vi "openOutput.vi"(8 "error in (no error)":errorcluster, 11 "DIO64Output in":refnum<class "DIO64Output.lvclass">) -> (0 "error out":errorcluster, 3 "DIO64Output out":refnum<class "DIO64Output.lvclass">)   [LabVIEW 2011, in "Hardware.lvlib" / "Channels.lvlib" / "DIO64Output.lvclass"]
doc: "Abstract Method.\n\nShould be overwritten by implementation of a digital output channel which require special treatment to initialise the channel.\n\nFor example, the Dio64 card require it to be opened and loaded, and kept in this state the whole time it is in use."
uses:
  DIO64Output.lvclass
  DIO64Output.lvclass/DIO64Output.ctl
  Channels.lvlib
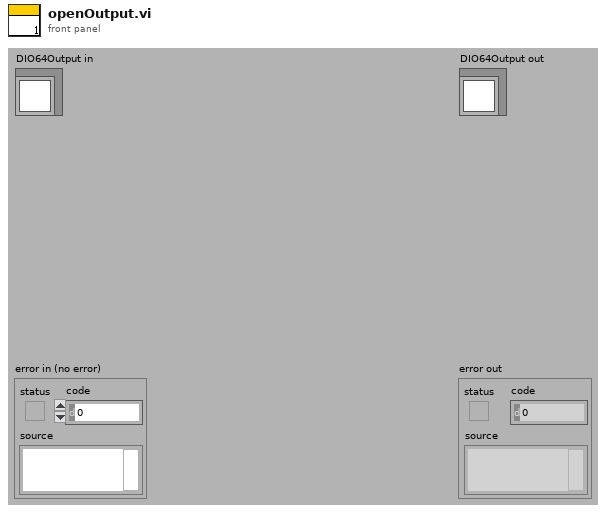
[diagram p1: front panel]
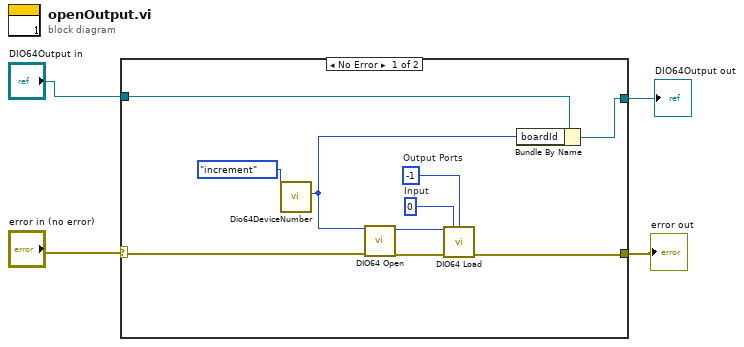
[diagram p0: block diagram]
diagram:
  n1 = case shown="No Error" "error in (no error)" {
    selector: "error in (no error)" -> [w9 w15]
    tunnel: "DIO64Output in" -> [w8 w16]
    tunnel: [w7 w16] -> w2
    tunnel: [w5 w15] -> w1
    frame No Error {
      w11 = -1  # Output Ports
      w12 = 0  # Input
      n2 = call "Dio64DeviceNumber.vi"("Action"=enum16{"increment", "deincrement"}."increment") -> ("Numeric"=w6:i32)  [unwired: 10 in]
      n3 = call <userlib>:"DIO64 Open.vi"("board in"=w6, "error in (no error)"=w9) -> ("board out"=w14:u16, "error out"=w13:errorcluster)  [unwired: 12 in]
      n4 = call <userlib>:"DIO64 Load.vi"("board in"=w14, "input hint"=w12, "output hint"=w11, "error in (no error)"=w13) -> ("error out"=w5:errorcluster)  [unwired: 10 in, 1 out]
      n5 = Bundle By Name(cluster=w8, "boardId"=w6) -> (w7:refnum<class "DIO64Output.lvclass">)
    }
    frame Error {
    }
  }
  "error out" <- w1
  "DIO64Output out" <- w2
